vi "STOP.vi"(11 "Class 2.lvclass":refnum<class "Class 2.lvclass">) -> (3 "Class 2.lvclass 2":refnum<class "Class 2.lvclass">)   [LabVIEW 2019, in "Class 2.lvclass"]
uses:
  Class 2.lvclass
  Class 2.lvclass/Class 2.ctl
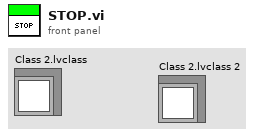
[diagram p1: front panel]
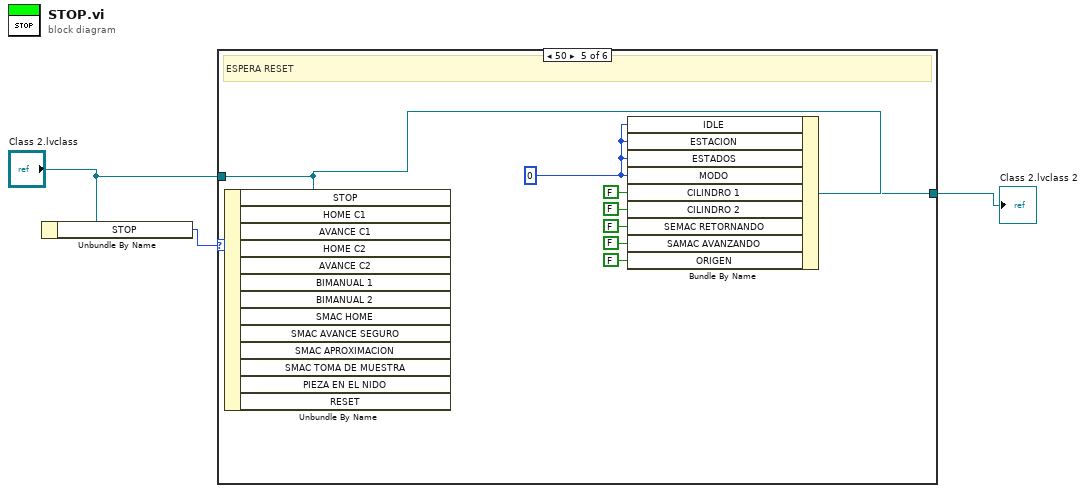
[diagram p0: block diagram]
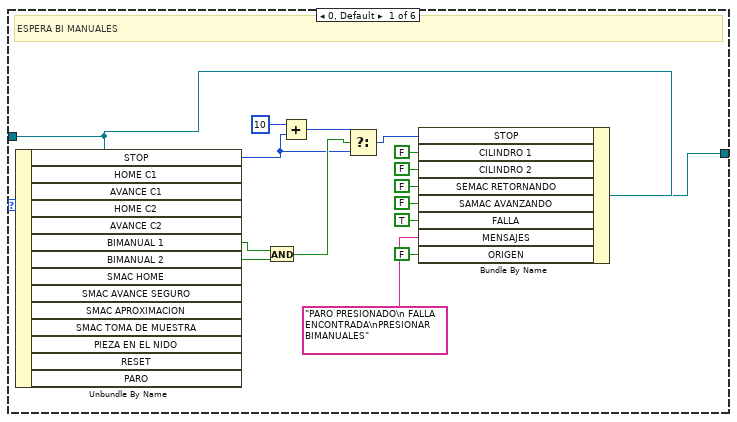
[diagram p2: hidden frame]
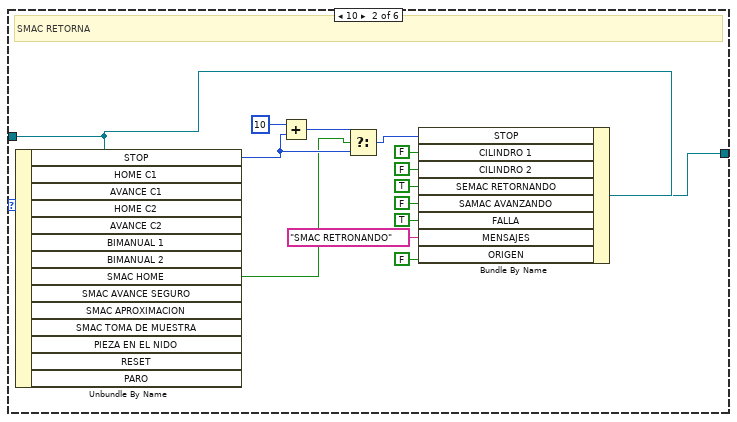
[diagram p3: hidden frame]
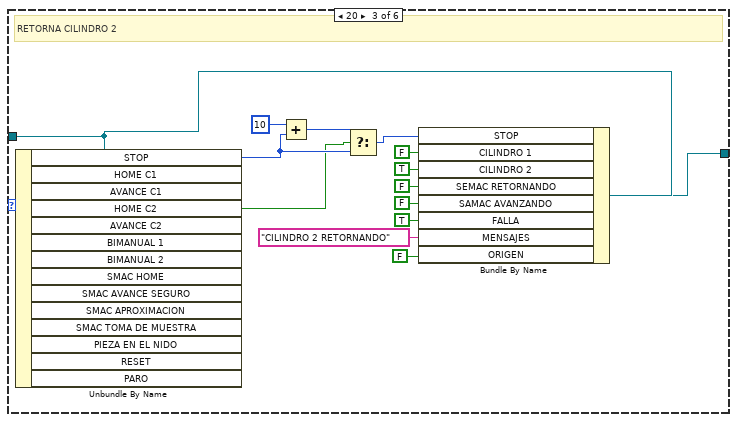
[diagram p4: hidden frame]
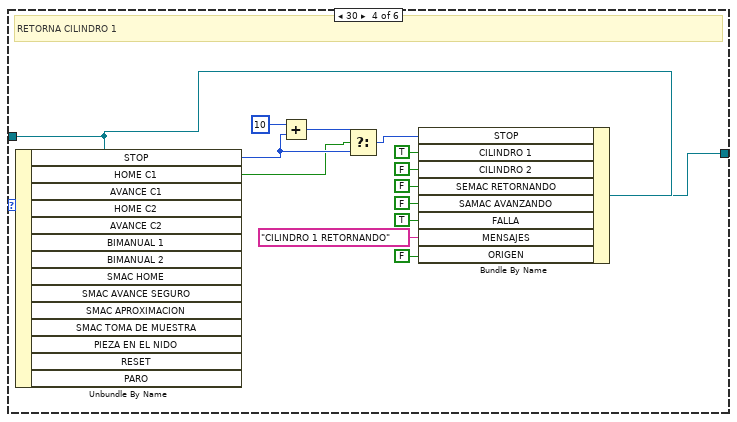
[diagram p5: hidden frame]
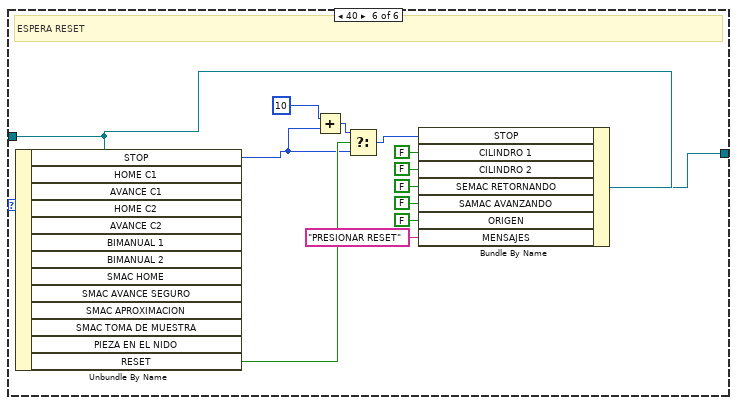
[diagram p6: hidden frame]
diagram:
  n1 = Unbundle By Name("Class 2.lvclass") -> ("STOP"=w3:i16)
  n2 = case shown="50" w3 {
    tunnel: "Class 2.lvclass" -> [w18 w32 w46 w60 w69 w82]
    tunnel: [w17 w31 w45 w59 w68 w81] -> w1
    frame 0, Default {
      # "ESPERA BI MANUALES"
      n3 = Unbundle By Name(w18) -> ("STOP"=w11:i16, "BIMANUAL 1"=w14:bool, "BIMANUAL 2"=w13:bool)  [unwired: 11 out]
      n4 = And(x=w14, y=w13) -> (x .and. y?=w12:bool)
      n5 = Add(x=i16 10, y=w11) -> (x+y=w16:i16)
      n6 = Select(t=w16, s=w12, f=w11) -> (s? t:f=w15:i16)
      n7 = Bundle By Name(cluster=w18, "STOP"=w15, "CILINDRO 1"=FALSE ("SALIDAS.CILINDRO 1"), "CILINDRO 2"=FALSE ("SALIDAS.CILINDRO 2"), "SEMAC RETORNANDO"=FALSE ("SALIDAS.SEMAC RETORNANDO"), "SAMAC AVANZANDO"=FALSE ("SALIDAS.SAMAC AVANZANDO"), "FALLA"=TRUE ("PROCESO.FALLA"), "MENSAJES"="PARO PRESIONADO\n FALLA ENCONTRADA\nPRESIONAR BIMANUALES" ("SALIDAS.MENSAJES"), "ORIGEN"=FALSE ("PROCESO.ORIGEN")) -> (w17:refnum<class "Class 2.lvclass">)
    }
    frame 10 {
      # "SMAC RETORNA"
      n8 = Unbundle By Name(w32) -> ("STOP"=w28:i16, "SMAC HOME"=w23:bool)  [unwired: 12 out]
      n9 = Add(x=i16 10, y=w28) -> (x+y=w30:i16)
      n10 = Select(t=w30, s=w23, f=w28) -> (s? t:f=w29:i16)
      n11 = Bundle By Name(cluster=w32, "STOP"=w29, "CILINDRO 1"=FALSE ("SALIDAS.CILINDRO 1"), "CILINDRO 2"=FALSE ("SALIDAS.CILINDRO 2"), "SEMAC RETORNANDO"=TRUE ("SALIDAS.SEMAC RETORNANDO"), "SAMAC AVANZANDO"=FALSE ("SALIDAS.SAMAC AVANZANDO"), "FALLA"=TRUE ("PROCESO.FALLA"), "MENSAJES"="SMAC RETRONANDO" ("SALIDAS.MENSAJES"), "ORIGEN"=FALSE ("PROCESO.ORIGEN")) -> (w31:refnum<class "Class 2.lvclass">)
    }
    frame 20 {
      # "RETORNA CILINDRO 2"
      n12 = Unbundle By Name(w46) -> ("STOP"=w42:i16, "HOME C2"=w37:bool)  [unwired: 12 out]
      n13 = Add(x=i16 10, y=w42) -> (x+y=w44:i16)
      n14 = Select(t=w44, s=w37, f=w42) -> (s? t:f=w43:i16)
      n15 = Bundle By Name(cluster=w46, "STOP"=w43, "CILINDRO 1"=FALSE ("SALIDAS.CILINDRO 1"), "CILINDRO 2"=TRUE ("SALIDAS.CILINDRO 2"), "SEMAC RETORNANDO"=FALSE ("SALIDAS.SEMAC RETORNANDO"), "SAMAC AVANZANDO"=FALSE ("SALIDAS.SAMAC AVANZANDO"), "FALLA"=TRUE ("PROCESO.FALLA"), "MENSAJES"="CILINDRO 2 RETORNANDO" ("SALIDAS.MENSAJES"), "ORIGEN"=FALSE ("PROCESO.ORIGEN")) -> (w45:refnum<class "Class 2.lvclass">)
    }
    frame 30 {
      # "RETORNA CILINDRO 1"
      n16 = Unbundle By Name(w60) -> ("STOP"=w56:i16, "HOME C1"=w51:bool)  [unwired: 12 out]
      n17 = Add(x=i16 10, y=w56) -> (x+y=w58:i16)
      n18 = Select(t=w58, s=w51, f=w56) -> (s? t:f=w57:i16)
      n19 = Bundle By Name(cluster=w60, "STOP"=w57, "CILINDRO 1"=TRUE ("SALIDAS.CILINDRO 1"), "CILINDRO 2"=FALSE ("SALIDAS.CILINDRO 2"), "SEMAC RETORNANDO"=FALSE ("SALIDAS.SEMAC RETORNANDO"), "SAMAC AVANZANDO"=FALSE ("SALIDAS.SAMAC AVANZANDO"), "FALLA"=TRUE ("PROCESO.FALLA"), "MENSAJES"="CILINDRO 1 RETORNANDO" ("SALIDAS.MENSAJES"), "ORIGEN"=FALSE ("PROCESO.ORIGEN")) -> (w59:refnum<class "Class 2.lvclass">)
    }
    frame 50 {
      w62 = i16 0 ("MAQ DE ESTADOS.MODO")
      # "ESPERA RESET"
      n20 = Unbundle By Name(w69) -> ()  [unwired: 13 out]
      n21 = Bundle By Name(cluster=w69, "IDLE"=w62, "ESTACION"=w62, "ESTADOS"=w62, "MODO"=w62, "CILINDRO 1"=FALSE ("SALIDAS.CILINDRO 1"), "CILINDRO 2"=FALSE ("SALIDAS.CILINDRO 2"), "SEMAC RETORNANDO"=FALSE ("SALIDAS.SEMAC RETORNANDO"), "SAMAC AVANZANDO"=FALSE ("SALIDAS.SAMAC AVANZANDO"), "ORIGEN"=FALSE ("PROCESO.ORIGEN")) -> (w68:refnum<class "Class 2.lvclass">)
    }
    frame 40 {
      # "ESPERA RESET"
      n22 = Unbundle By Name(w82) -> ("STOP"=w71:i16, "RESET"=w75:bool)  [unwired: 11 out]
      n23 = Add(x=i16 10 ("t"), y=w71) -> (x+y=w70:i16)
      n24 = Select(t=w70, s=w75, f=w71) -> (s? t:f=w73:i16)
      n25 = Bundle By Name(cluster=w82, "STOP"=w73, "CILINDRO 1"=FALSE ("SALIDAS.CILINDRO 1"), "CILINDRO 2"=FALSE ("SALIDAS.CILINDRO 2"), "SEMAC RETORNANDO"=FALSE ("SALIDAS.SEMAC RETORNANDO"), "SAMAC AVANZANDO"=FALSE ("SALIDAS.SAMAC AVANZANDO"), "ORIGEN"=FALSE ("PROCESO.ORIGEN"), "MENSAJES"="PRESIONAR RESET" ("SALIDAS.MENSAJES")) -> (w81:refnum<class "Class 2.lvclass">)
    }
  }
  "Class 2.lvclass 2" <- w1
